vi "Set value and frequency.vi"(7 "Ignore instr. error (false)":bool, 8 "error in":errorcluster, 9 "Frequency [Hz]":dbl=10.0 min=10.0 max=1000000.0, 10 "Value":dbl, 11 "VISA resource name":refnum<visa-resource-name>) -> (0 "error out":errorcluster, 2 "Setup failed":bool, 3 "VISA resource name out":refnum<visa-resource-name>)   [LabVIEW 2013, in "Datron D4xxx.lvlib"]
doc: "This VI sets value and frequency at once. Parameters are same as in set value/frequency VIs."
uses:
  Datron D4xxx.lvlib
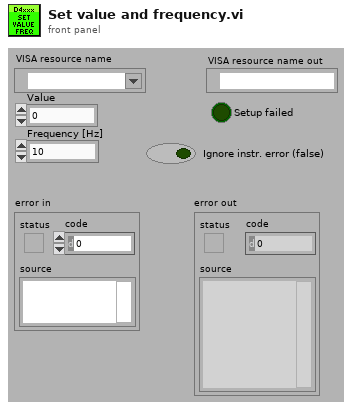
[diagram p1: front panel]
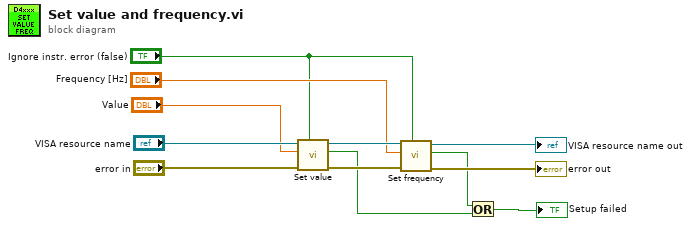
[diagram p0: block diagram]
diagram:
  n1 = call "Set value.vi"("Ignore range overflow error (false)"="Ignore instr. error (false)", "error in"="error in", "Value"="Value", "VISA resource name"="VISA resource name") -> ("error out"=w9:errorcluster, "Set value failed"=w2:bool, "VISA resource name out"=w10:refnum<visa-resource-name>)  [unwired: 5 in]
  n2 = call "Set frequency.vi"("Ignore out of range error (false)"="Ignore instr. error (false)", "error in"=w9, "Frequency"="Frequency [Hz]", "VISA resource name"=w10) -> ("error out"=→"error out":errorcluster, "Set frequency failed"=w3:bool, "VISA resource name out"=→"VISA resource name out":refnum<visa-resource-name>)  [unwired: 5 in]
  n3 = Or(x=w3, y=w2) -> (x .or. y?=→"Setup failed":bool)
